vi "Read Numeric Parameters from string.vi"(11 "String":string) -> (3 "Parameters - numeric":T1[](array[typedef]))   [LabVIEW 2020, in "Run Utilities.lvlib" / "Optimiser Cell.lvclass"]
uses:
  Optimiser Cell.lvclass
  Optimise parameter - numeric.ctl
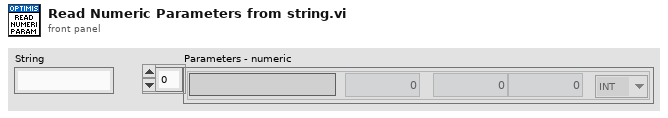
[diagram p1: front panel]
types:
  T1 = typedef "Run Utilities.lvlib/Optimiser Cell.lvclass/Optimise parameter - numeric.ctl" = cluster{"Name":string, "Start value":dbl, "From":dbl, "To":dbl, "dtype":enum16{"INT", "DBL"}}
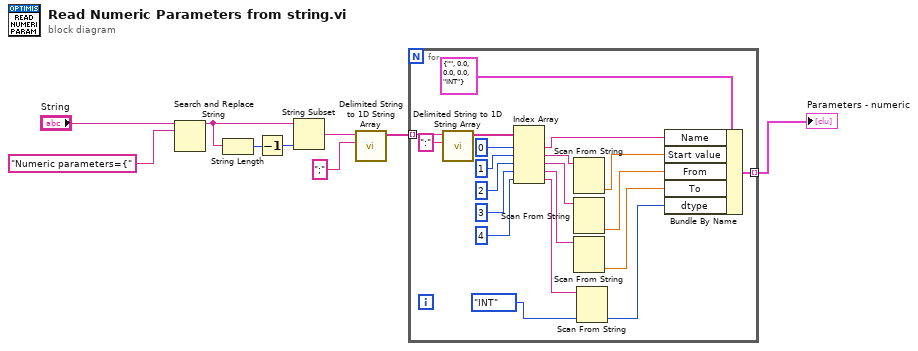
[diagram p0: block diagram]
diagram:
  n1 = Search and Replace String(input string="String", search string="Numeric parameters={") -> (result string=w8:string)  [unwired: 6 in, 3 out]
  n2 = String Length(string=w8) -> (length=w7:i32)
  n3 = Decrement(x=w7) -> (x-1=w6:i32)
  n4 = String Subset(string=w8, length (rest)=w6) -> (substring=w5:string)  [unwired: 1 in]
  n5 = call <vilib>:"Delimited String to 1D String Array.vi"("delimiter"=";", "delimited string"=w5) -> ("string array"=w3:string[])  [unwired: 9 in]
  n6 = for {
    tunnel: w3 -> [w29] mode=indexing
    tunnel: [w23] -> w1 mode=indexing
    n7 = call <vilib>:"Delimited String to 1D String Array.vi"("delimiter"=":", "delimited string"=w29) -> ("string array"=w20:string[])  [unwired: 9 in]
    n8 = Index Array(array=w20, index #1=0 ("index"), index #2=1 ("index"), index #3=2 ("index"), index #4=3 ("index"), index #5=4 ("index")) -> (element #1=w27:string, element #2=w14:string, element #3=w13:string, element #4=w12:string, element #5=w11:string)
    n9 = Scan From String(input string=w14) -> (output 1=w24:dbl)  [unwired: 4 in, 3 out]
    n10 = Scan From String(input string=w13) -> (output 1=w25:dbl)  [unwired: 4 in, 3 out]
    n11 = Scan From String(input string=w12) -> (output 1=w26:dbl)  [unwired: 4 in, 3 out]
    n12 = Scan From String(input string=w11, default 1=enum16{"INT", "DBL"}."INT" ("dtype")) -> (output 1=w22:enum16{"INT", "DBL"})  [unwired: 3 in, 3 out]
    n13 = Bundle By Name(cluster=T1 {"Name"="", "Start value"=0.0, "From"=0.0, "To"=0.0, "dtype"=enum."INT"} ("Optimise parameter"), "Name"=w27, "Start value"=w24, "From"=w25, "To"=w26, "dtype"=w22) -> (w23:T1)
  }
  "Parameters - numeric" <- w1
